vi "0xEE_Read_device_description_fragment_in_JSON_format.vi"(8 "error in":errorcluster, 11 "paramUnicorn 2":T1={"conParam"={"ReadIntParam"=TRUE, "ReadDescrParam"=FALSE, "ReadFloatParam"=TRUE, "debug"=FALSE, "ReadJSON"=TRUE, "IP_address"="192.168.1.216", "N_attempts"=3, "type_con"=enum."TCP", "MB_address"=1, "VISA"="COM1", "connection ID"=refnum, "nameDevices"="", "timeout"=3000, "port"=2000, "type_version"="0F0C0001", "baud_rate"=115200, "VersionControl"=TRUE, "TCP_conn"=TRUE, "WindowSize"=700}, "Param"={"NumParam"={"NTelem"=201, "NInt"=16, "NFloat"=10, "NTable"=2}, "ParamInt"=[{"ID"="Режим работы", "Num"=0, "Name"="", "Type"="", "Enum"="", "Desc"="", "Unit"="", "Access"="", "FormatStr"="", "Min"=0, "Max"=0}, {"ID"="", "Num"=0, "Name"="", "Type"="", "Enum"="", "Desc"="", "Unit"="", "Access"="", "FormatStr"="", "Min"=0, "Max"=0}, {"ID"="", "Num"=0, "Name"="", "Type"="", "Enum"="", "Desc"="", "Unit"="", "Access"="", "FormatStr"="", "Min"=0, "Max"=0}, {"ID"="", "Num"=0, "Name"="", "Type"="", "Enum"="", "Desc"="", "Unit"="", "Access"="", "FormatStr"="", "Min"=0, "Max"=0}, {"ID"="", "Num"=0, "Name"="", "Type"="", "Enum"="", "Desc"="", "Unit"="", "Access"="", "FormatStr"="", "Min"=0, "Max"=0}, {"ID"="", "Num"=0, "Name"="", "Type"="", "Enum"="", "Desc"="", "Unit"="", "Access"="", "FormatStr"="", "Min"=0, "Max"=0}, {"ID"="ModeWork", "Num"=0, "Name"="", "Type"="", "Enum"="", "Desc"="", "Unit"="", "Access"="", "FormatStr"="", "Min"=0, "Max"=0}], "Telemetry"=[], "Table"=[], "ParamFloat"=[]}}) -> (0 "error out":errorcluster, 2 "JSONStr":string, 3 "paramUnicorn":T1={"conParam"={"ReadIntParam"=TRUE, "ReadDescrParam"=FALSE, "ReadFloatParam"=TRUE, "debug"=FALSE, "ReadJSON"=TRUE, "IP_address"="192.168.1.216", "N_attempts"=3, "type_con"=enum."TCP", "MB_address"=1, "VISA"="COM1", "connection ID"=refnum, "nameDevices"="", "timeout"=3000, "port"=2000, "type_version"="0F0C0001", "baud_rate"=115200, "VersionControl"=TRUE, "TCP_conn"=TRUE, "WindowSize"=700}, "Param"={"NumParam"={"NTelem"=201, "NInt"=16, "NFloat"=10, "NTable"=2}, "ParamInt"=[{"ID"="Режим работы", "Num"=0, "Name"="", "Type"="", "Enum"="", "Desc"="", "Unit"="", "Access"="", "FormatStr"="", "Min"=0, "Max"=0}, {"ID"="", "Num"=0, "Name"="", "Type"="", "Enum"="", "Desc"="", "Unit"="", "Access"="", "FormatStr"="", "Min"=0, "Max"=0}, {"ID"="", "Num"=0, "Name"="", "Type"="", "Enum"="", "Desc"="", "Unit"="", "Access"="", "FormatStr"="", "Min"=0, "Max"=0}, {"ID"="", "Num"=0, "Name"="", "Type"="", "Enum"="", "Desc"="", "Unit"="", "Access"="", "FormatStr"="", "Min"=0, "Max"=0}, {"ID"="", "Num"=0, "Name"="", "Type"="", "Enum"="", "Desc"="", "Unit"="", "Access"="", "FormatStr"="", "Min"=0, "Max"=0}, {"ID"="", "Num"=0, "Name"="", "Type"="", "Enum"="", "Desc"="", "Unit"="", "Access"="", "FormatStr"="", "Min"=0, "Max"=0}, {"ID"="ModeWork", "Num"=0, "Name"="", "Type"="", "Enum"="", "Desc"="", "Unit"="", "Access"="", "FormatStr"="", "Min"=0, "Max"=0}], "Telemetry"=[], "Table"=[], "ParamFloat"=[]}})   [LabVIEW 2017, in "LV_Unicorn.lvlib"]
uses:
  LV_Unicorn.lvlib
  Control/unicorn_Param.ctl
  Control/unicorn_conn.ctl
  Control/unicorn_JSON.ctl
  Control/unicorn_ParamInt.ctl
  Control/unicorn_Telemetry.ctl
  Control/unicorn_Table.ctl
  Control/unicorn_ParamFloat.ctl
panel:
  out "error out 2":errorcluster
  out "Slide 2":u8(slide) scale=0.0..100.0
  out "String out":string
  out "Смешение в байтах":i32
  out "Размер данных":i32
  out "Размер описания":i32
  out "Размер фрагмента":i32
  # "Чтение описания устройства"
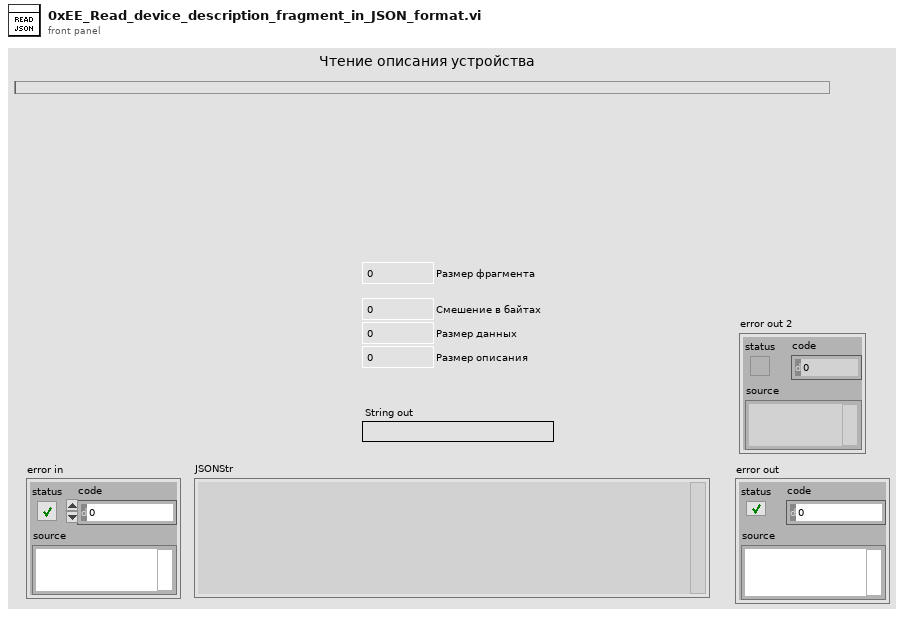
[diagram p1: front panel]
types:
  T1 = typedef "LV_Unicorn.lvlib/unicorn_Param.ctl" = cluster{"conParam":T2, "Param":T3}
  T2 = typedef "LV_Unicorn.lvlib/unicorn_conn.ctl" = cluster{"ReadIntParam":bool, "ReadDescrParam":bool, "ReadFloatParam":bool, "debug":bool, "ReadJSON":bool, "IP_address":string, "N_attempts":i32, "type_con":enum16{"Serial", "TCP"}, "MB_address":i32, "VISA":refnum<visa-resource-name>, "connection ID":refnum<k5>, "nameDevices":string, "timeout":i32, "port":u16, "type_version":string, "baud_rate":u32, "VersionControl":bool, "TCP_conn":bool, "WindowSize":i32}
  T3 = typedef "LV_Unicorn.lvlib/unicorn_JSON.ctl" = cluster{"NumParam":cluster{"NTelem":i32, "NInt":i32, "NFloat":i32, "NTable":i32}, "ParamInt":T4, "Telemetry":T5, "Table":T6, "ParamFloat":T7}
  T4 = typedef "LV_Unicorn.lvlib/unicorn_ParamInt.ctl" = cluster{"ID":string, "Num":i32, "Name":string, "Type":string, "Enum":string, "Desc":string, "Unit":string, "Access":string, "FormatStr":string, "Min":i32, "Max":i32}[]
  T5 = typedef "LV_Unicorn.lvlib/unicorn_Telemetry.ctl" = cluster{"ID":string, "Num":i32, "Name":string, "Desc":string, "Unit":string, "FormatStr":string, "Min":i32, "Max":i32}[]
  T6 = typedef "LV_Unicorn.lvlib/unicorn_Table.ctl" = cluster{"Num":i32, "Access":string, "ColumnCount":i32, "NeedParamPrepare":bool, "Columns":cluster{"Column":i32, "Desc":string, "Name":string}[], "DataType":string, "FormatStr":string, "ID":string, "Name":string, "RowCount":i32, "Rows":cluster{"Desc":string, "ID":string, "Max":i32, "Min":i32, "Name":string, "Row":i32, "Unit":string}[], "Type":string}[]
  T7 = typedef "LV_Unicorn.lvlib/unicorn_ParamFloat.ctl" = cluster{"ID":string, "Num":i32, "Name":string, "Type":string, "Enum":string, "Desc":string, "Unit":string, "Access":string, "FormatStr":string, "Min":sgl, "Max":sgl}[]
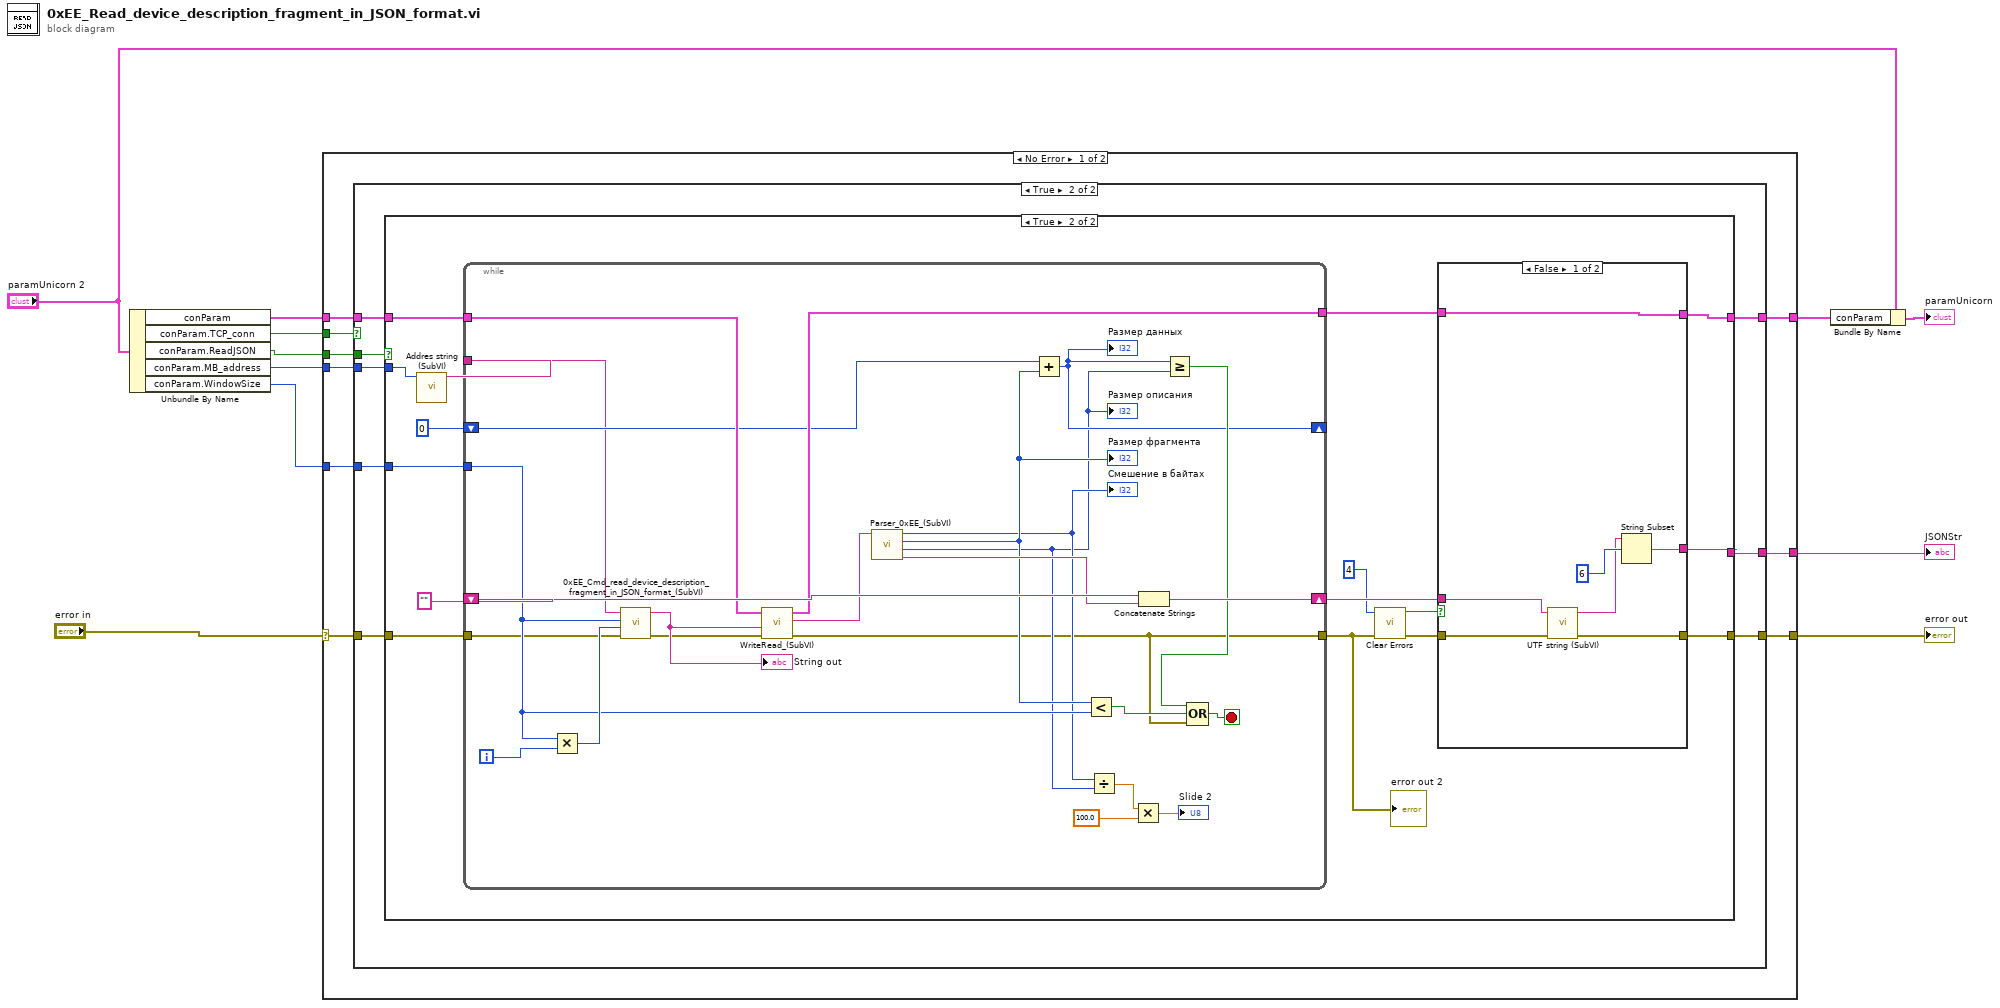
[diagram p0: block diagram]
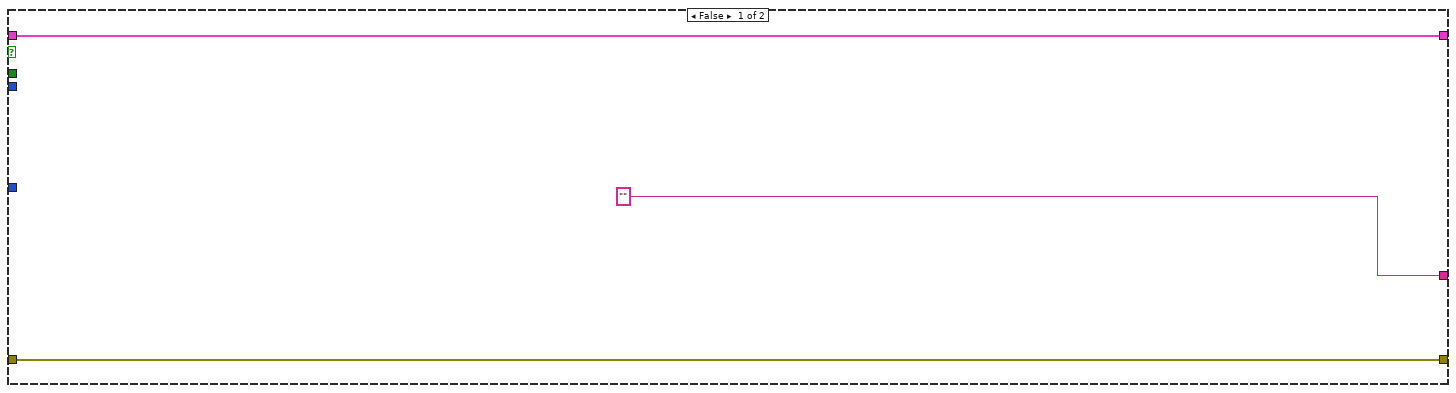
[diagram p2: hidden frame]
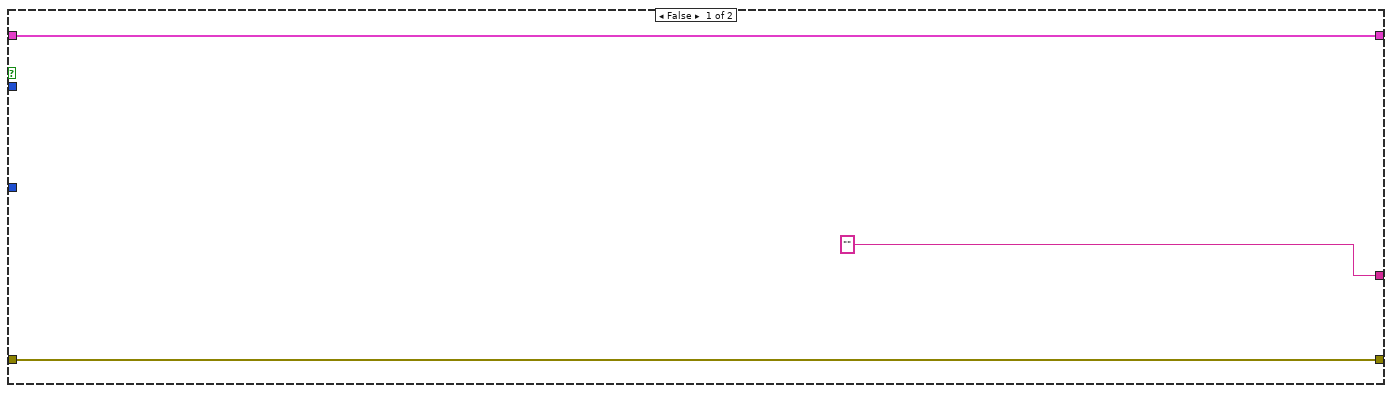
[diagram p3: hidden frame]
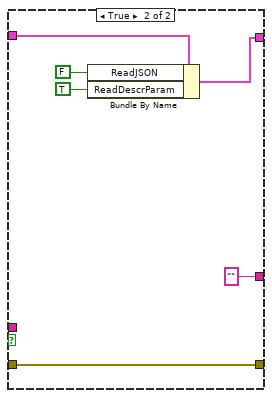
[diagram p4: hidden frame]
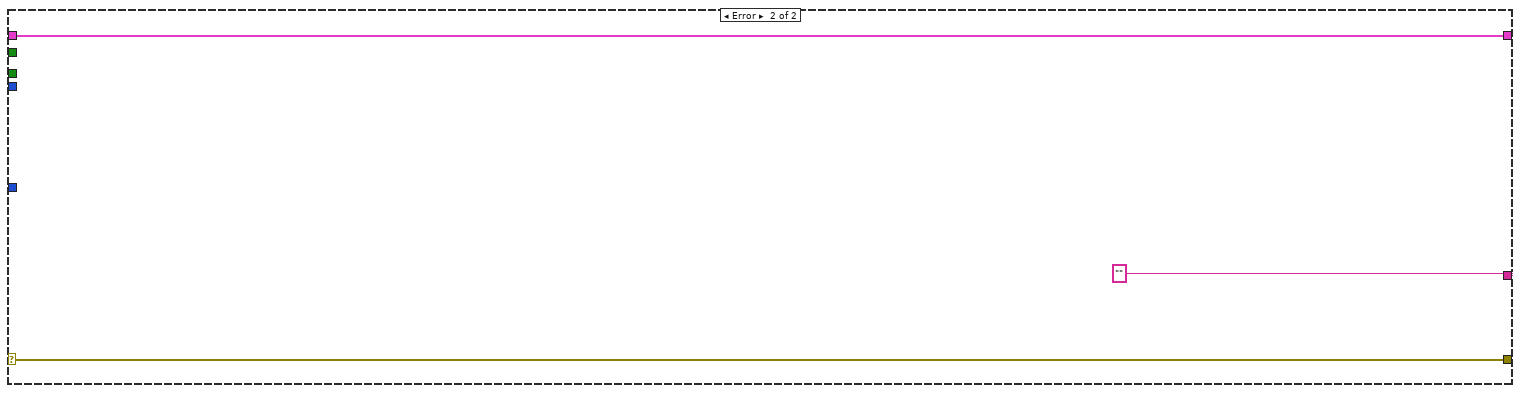
[diagram p5: hidden frame]
diagram:
  n1 = Unbundle By Name("paramUnicorn 2") -> ("conParam"=w5:T2, "conParam.TCP_conn"=w4:bool, "conParam.ReadJSON"=w3:bool, "conParam.MB_address"=w2:i32, "conParam.WindowSize"=w1:i32)
  n2 = case shown="No Error" "error in" {
    selector: "error in" -> [w17 w91]
    tunnel: [w20 w90] -> w8
    tunnel: w5 -> [w16 w90]
    tunnel: [w19 w91] -> w11
    tunnel: [w18 "" ("StringOut")] -> w10
    tunnel: w4 -> [w15 _]
    tunnel: w3 -> [w14 _]
    tunnel: w2 -> [w13 _]
    tunnel: w1 -> [w12 _]
    frame No Error {
      n3 = case shown="True" w15 {
        tunnel: [w22 w31] -> w20
        tunnel: [w23 w30] -> w19
        tunnel: ["" ("StringOut") w29] -> w18
        tunnel: w17 -> [w23 w28]
        tunnel: w16 -> [w22 w27]
        tunnel: w14 -> [_ w26]
        tunnel: w13 -> [_ w25]
        tunnel: w12 -> [_ w24]
        frame False {
        }
        frame True {
          n4 = case shown="True" w26 {
            tunnel: [w34 w36] -> w31
            tunnel: w27 -> [w34 w48]
            tunnel: [w33 w38] -> w30
            tunnel: ["" ("StringOut") w45] -> w29
            tunnel: w28 -> [w33 w44]
            tunnel: w25 -> [_ w43]
            tunnel: w24 -> [_ w42]
            frame False {
            }
            frame True {
              n5 = call "Addres string (SubVI).vi"("Адрес"=w43) -> ("String"=w46:string)  [unwired: 10 in]
              n6 = while {
                shift-right: [w83] -> w49
                shift-left: "" ("substring") -> [w85]
                tunnel: w48 -> [w80]
                tunnel: [w79] -> w37
                tunnel: w44 -> [w65]
                tunnel: [w64] -> w35
                shift-right: [w76] -> _
                shift-left: 0 -> [w75]
                tunnel: w46 -> [w74]
                tunnel: w42 -> [w73]
                i -> [w87]
                stop <- w81 stop-if-true
                n7 = Multiply(x=w73, y=w87) -> (x*y=w86:i32)
                n8 = call "0xEE_Cmd_read_device_description_fragment_in_JSON_format_(SubVI).vi"("error in"=w65, "Смешение в байтах"=w86, "Макс размер"=w73, "String in"=w74) -> ("error out"=w66:errorcluster, "String out"=w88:string)  [unwired: 6 in]
                "String out" <- w88
                n9 = call "WriteRead_(SubVI).vi"("error in"=w66, "Запрос"=w88, "ParamIn"=w80) -> ("error out"=w64:errorcluster, "Ответ"=w72:string, "ParamOut"=w79:T2)  [unwired: 4 in, 2 out]
                n10 = call "Parser_0xEE_(SubVI).vi"("String in"=w72) -> ("substring"=w84:string, "Размер описания"=w70:i32, "Размер фрагмента"=w82:i32, "Смешение в байтах"=w71:i32)  [unwired: 7 in]
                "Смешение в байтах" <- w71
                "Размер описания" <- w70
                "Размер фрагмента" <- w82
                n11 = Add(x=w75, y=w82) -> (x+y=w76:i32)
                "Размер данных" <- w76
                n12 = Less?(x=w82, y=w73) -> (x < y?=w78:bool)
                n13 = Divide(x=w71, y=w70) -> (x/y=w69:dbl)
                n14 = Multiply(x=w69, y=100.0) -> (x*y=→"Slide 2":dbl)
                n15 = Concatenate Strings(w85, w84) -> (w83:string)
                n16 = Greater Or Equal?(x=w76, y=w70) -> (x >= y?=w77:bool)
                n17 = Compound Arithmetic op=OR(w77, w78, w64) -> (w81:bool)
              }
              "error out 2" <- w35
              n18 = call <vilib>:"Clear Errors.vi"("error in (no error)"=w35, "specific error code to clear (0: all)"=4) -> ("error out"=w40:errorcluster, "specific error cleared?"=w39:bool)  [unwired: 4 in]
              n19 = case shown="False" w39 {
                tunnel: w49 -> [w57 _]
                tunnel: [w54 "" ("StringOut")] -> w45
                tunnel: w40 -> [w53 w63]
                tunnel: [w52 w63] -> w38
                tunnel: w37 -> [w51 w60]
                tunnel: [w51 w59] -> w36
                frame False {
                  n20 = call "UTF string (SubVI).vi"("error in"=w53, "StringIn"=w57) -> ("error out"=w52:errorcluster, "StringOut"=w55:string)  [unwired: 8 in]
                  n21 = String Subset(string=w55, offset (0)=6) -> (substring=w54:string)  [unwired: 1 in]
                }
                frame True {
                  n22 = Bundle By Name(cluster=w60, "ReadJSON"=FALSE, "ReadDescrParam"=TRUE) -> (w59:T2)
                }
              }
            }
          }
        }
      }
    }
    frame Error {
    }
  }
  "JSONStr" <- w10
  "error out" <- w11
  n23 = Bundle By Name(cluster="paramUnicorn 2", "conParam"=w8) -> (→"paramUnicorn":T1)
